vi "Load Control Panel VI.vi"(8 "error in (no error)":errorcluster, 11 "Device":refnum<class "Device.lvclass">) -> (0 "error out":errorcluster, 2 "vi ref out":refnum<vi>, 3 "Device out":refnum<class "Device.lvclass">)   [LabVIEW 2015, in "Device.lvclass"]
uses:
  Device.lvclass
  Device.lvclass/Device.ctl
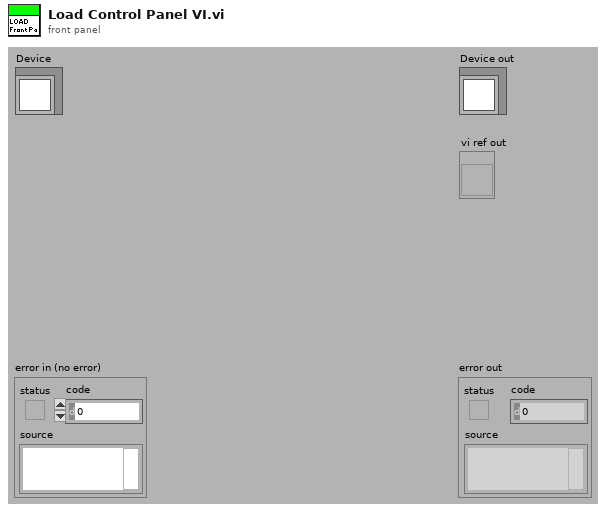
[diagram p1: front panel]
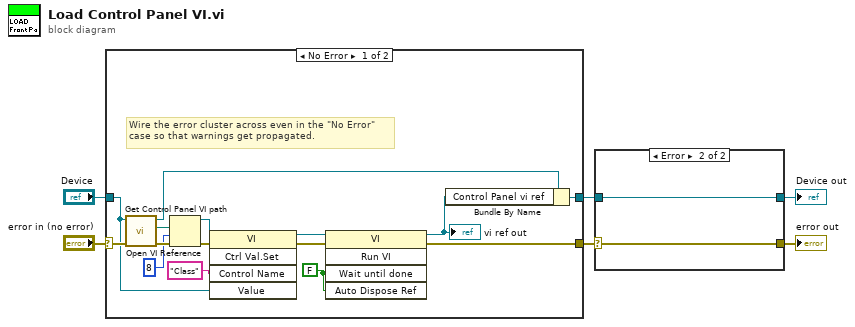
[diagram p0: block diagram]
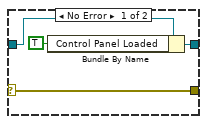
[diagram p2: hidden frame]
diagram:
  n1 = case shown="No Error" "error in (no error)" {
    selector: "error in (no error)" -> [w21 w23]
    tunnel: [w17 w23] -> w6
    tunnel: [w9 w22] -> w5
    tunnel: "Device" -> [w18 w22]
    frame No Error {
      w16 = FALSE ("Wait Until Done")
      # "Wire the error cluster across even in the \"No Error\"\ncase so that warnings get propagated."
      n2 = call-dynamic "Get Control Panel VI path.vi"("error in (no error)"=w21, "Device in"=w18) -> ("error out"=w19:errorcluster, "Control Panel VI path"=w20:path, "Device out"=w10:refnum<class "Device.lvclass">)  [unwired: 7 in]
      n3 = Open VI Reference(vi path=w20, options=8, error in (no error)=w19) -> (vi reference=w11:refnum<vi>, error out=w13:errorcluster)  [unwired: 3 in]
      n4 = invoke class="VI" method="Ctrl Val.Set"(reference=w11, error in=w13, "Control Name"="Class", "Value"=w18) -> (reference out=w7:refnum<vi>, error out=w15:errorcluster)  [unwired: 1 in, 3 out]
      n5 = invoke class="VI" method="Run VI"(reference=w7, error in=w15, "Wait until done"=w16, "Auto Dispose Ref"=w16) -> (reference out=w8:refnum<vi>, error out=w17:errorcluster)  [unwired: 1 in, 3 out]
      "vi ref out" <- w8
      n6 = Bundle By Name(cluster=w10, "Control Panel vi ref"=w8) -> (w9:refnum<class "Device.lvclass">)
    }
    frame Error {
    }
  }
  n7 = case shown="Error" w6 {
    selector: w6 -> [w24 w28]
    tunnel: w5 -> [w27 w29]
    tunnel: [w26 w29] -> w1
    tunnel: [w24 w28] -> w2
    frame No Error {
      n8 = Bundle By Name(cluster=w27, "Control Panel Loaded"=TRUE ("Front Panel Loaded")) -> (w26:refnum<class "Device.lvclass">)
    }
    frame Error {
    }
  }
  "error out" <- w2
  "Device out" <- w1
